vi "Init Device.vi"(8 "error in (no error)":errorcluster, 11 "Toggle 8 in":refnum<class "Toggle 8.lvclass">) -> (0 "error out":errorcluster, 3 "Toggle 8 out":refnum<class "Toggle 8.lvclass">)   [LabVIEW 2020, in "Toggle 8.lvclass"]
doc: "Init the device com port.\nThis should be called by the child class and the child class is responsible for setting the device as its default state."
uses:
  Toggle 8.lvclass
  C:/Sandbox/RF Bench/Source Code/WiSpry Test Framework/Devices/Device.lvclass
  PIC-device/PIC-Device.lvclass
  <instrlib>/Keithley 24XX/Keithley 24XX.lvlib
panel:
  out "Horizontal Graduated Bar":u8(slide) scale=0.0..100.0
  out "Cycle":i32=1
  in  "Stop Button":bool
  # "Beam cycling"
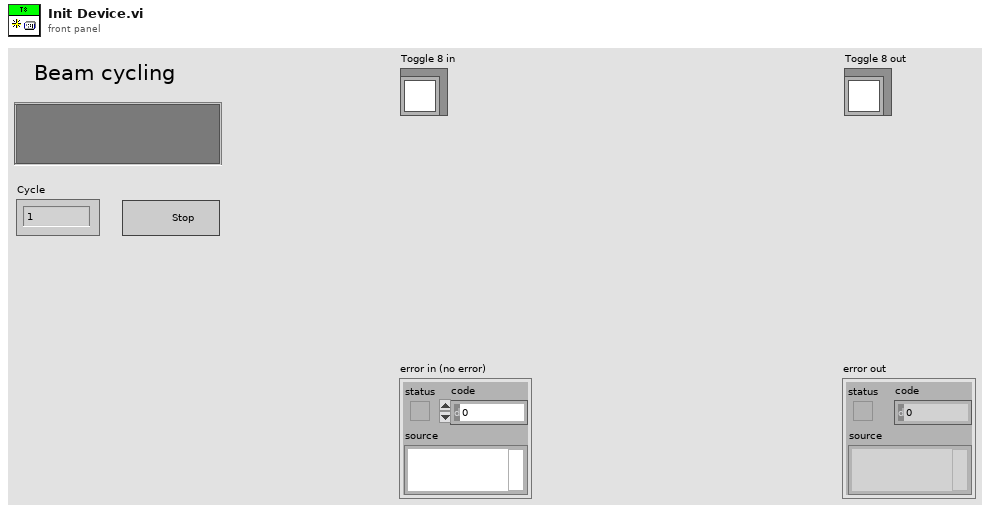
[diagram p1: front panel]
types:
  T1 = enum16{"RFFE 2-wire", "WiSPI 3-wire spi_sel", "WiSPI 4-wire spi_sel", "ifxSPI 3-wire spi_sel", "WiSPI 3-wire dev add spi_sel"}
  T2 = typedef "PIC-Device.lvclass/Register to Write.ctl" = cluster{"Register":u32, "Value":u32, "Dev Address":u32, "Physical Adress":u32}
  T3 = typedef "Toggle 8.lvclass/Test Sequence.ctl" = cluster{"CP values":string, "Charge Pump values":enum16{"CP 24V", "CP 26V", "CP 28V", "CP 30V", "CP 31V", "CP 32V", "CP 33V", "CP 34V", "CP 35V", "CP 36V", "CP 37V", "CP 38V", "CP 39V", "CP 40V", "CP 41V", "CP 42V", "CP 43V", "CP 44V", "CP 45V", "CP 46V", "CP 47V", "CP 48V", "CP 49V", "CP 50V", "CP 51V", "CP 52V", "CP 53V", "CP 54V", "CP 56V", "CP 58V", "CP 60V", "CP 62V"}[], "Charge Pump":T2[], "Control individual beams":bool, "OTP/beam values":dbl[], "Capa settings":T2[], "OTP Values string":string}
  T4 = typedef "Device.lvclass/Device Information Cluster.ctl" = cluster{"Device Info":string[][], "Default Values":T2[], "Fetched info":string[][]}
  T5 = cluster{"Enable":bool, "User init values":string}
  T6 = cluster{"Cycle":bool, "Number of cycles":u32, "Cycles Executed":u32}
  T7 = enum32{"Invalid", "Standard", "Closed", "Hidden", "Minimized", "Maximized"}
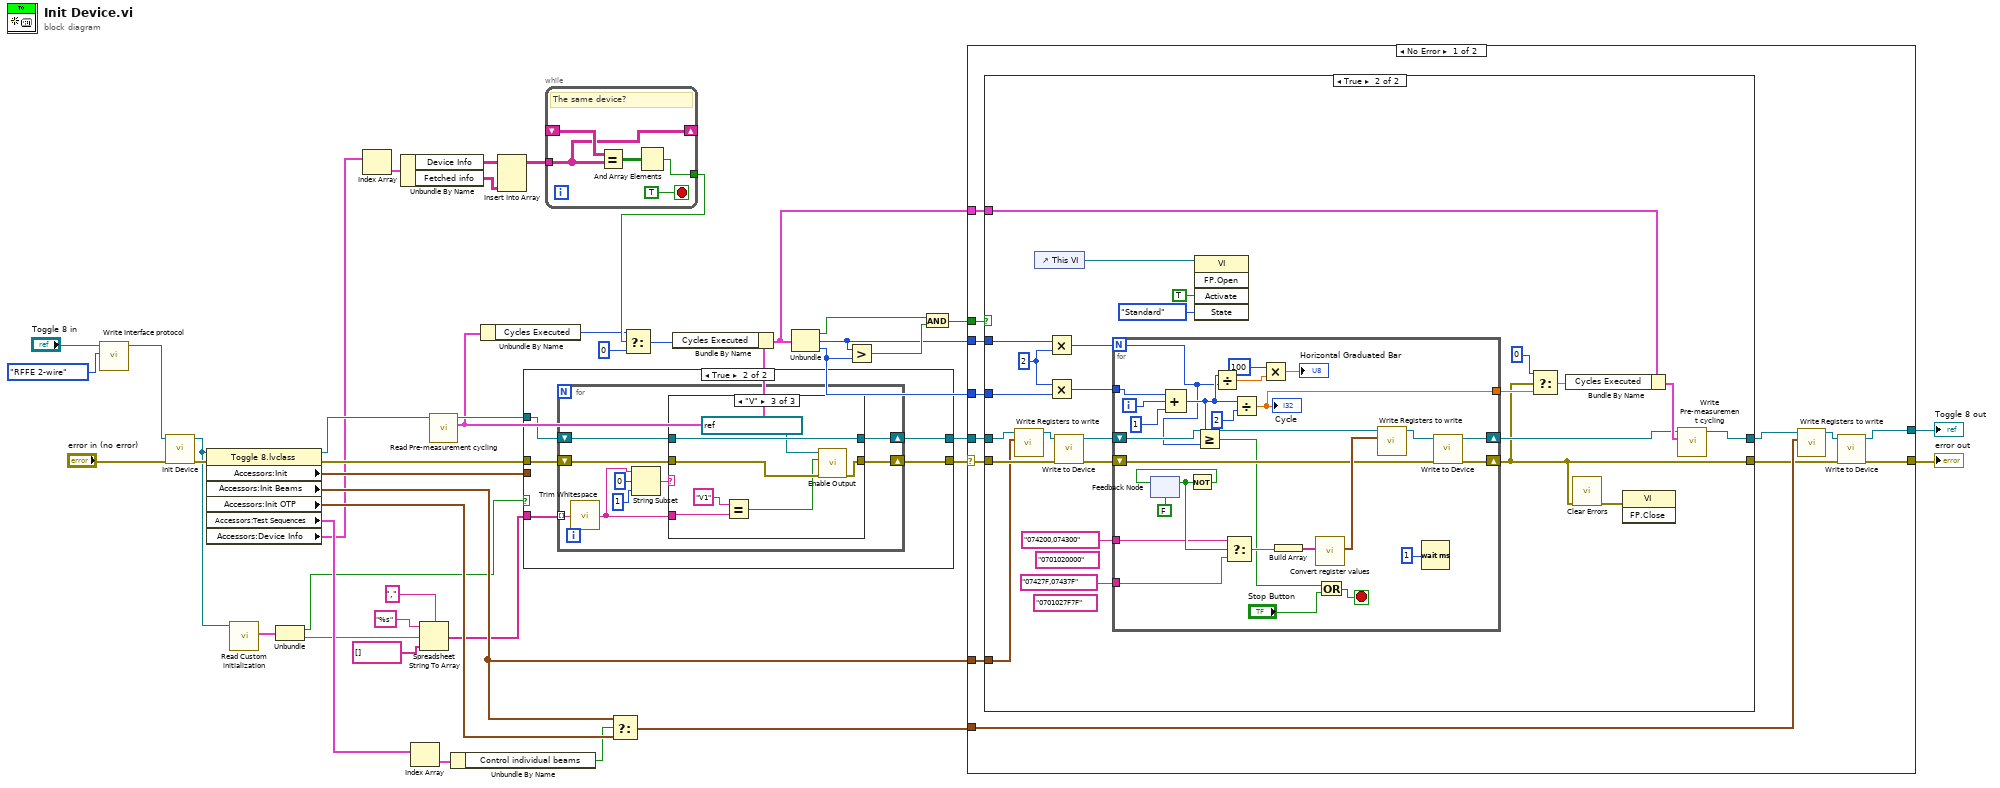
[diagram p0: block diagram]
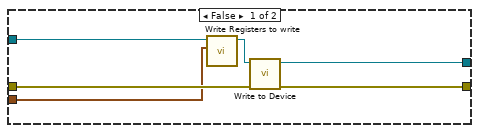
[diagram p2: hidden frame]
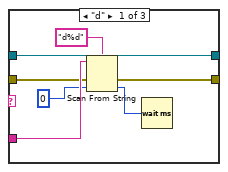
[diagram p3: hidden frame]
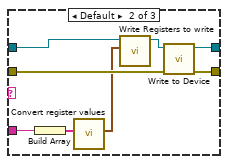
[diagram p4: hidden frame]
diagram:
  n1 = call-dynamic "Write Interface protocol.vi"("Interface protocol"=T1."RFFE 2-wire", "Device in"="Toggle 8 in") -> ("Device out"=w40:refnum<class "Toggle 8.lvclass">)  [unwired: 9 in]
  n2 = call-parent "Init Device.vi"("error in (no error)"="error in (no error)", "Device in"=w40) -> ("error out"=w38:errorcluster, "Device out"=w8:refnum<class "Toggle 8.lvclass">)  [unwired: 8 in]
  n3 = property class="Toggle 8.lvclass"(reference=w8, error in=w38) -> (reference out=w34:refnum<class "Toggle 8.lvclass">, error out=w39:errorcluster, "Accessors:Init"=w26:T2[], "Accessors:Init Beams"=w25:T2[], "Accessors:Init OTP"=w35:T2[], "Accessors:Test Sequences"=w37:T3[], "Accessors:Device Info"=w19:T4[])
  n4 = call-dynamic "Read Custom initialization.vi"("Toggle 8 in"=w8) -> ("Custom initialization"=w7:T5)  [unwired: 9 in, 1 out]
  n5 = Unbundle(w7) -> ("Enable"=w2:bool, "User init values"=w6:string)
  n6 = Index Array(array=w19) -> (element=w18:T4)  [unwired: 1 in]
  n7 = Unbundle By Name(w18) -> ("Device Info"=w11:string[][], "Fetched info"=w9:string[][])
  n8 = Index Array(array=w37) -> (element=w36:T3)  [unwired: 1 in]
  n9 = Spreadsheet String To Array(delimiter (Tab)=",", format string="%s", spreadsheet string=w6, array type (2D Dbl)=string[] []) -> (array=w1:string[])
  n10 = call-dynamic "Read Pre-measurement cycling.vi"("PIC-Device in"=w34) -> ("Pre-measurement cycling"=w16:T6, "PIC-Device out"=w33:refnum<class "Toggle 8.lvclass">)  [unwired: 9 in]
  n11 = Unbundle By Name(w36) -> ("Control individual beams"=w32:bool)
  n12 = Unbundle By Name(w16) -> ("Cycles Executed"=w14:u32)
  n13 = Insert Into Array(array=w11, new element=w9) -> (w10:string[][])  [unwired: 2 in]
  n14 = case shown="True" w2 {
    tunnel: w39 -> [w48 w54]
    tunnel: w33 -> [w47 w53]
    tunnel: [w46 w52] -> w31
    tunnel: [w45 w51] -> w30
    tunnel: w26 -> [w44 _]
    tunnel: w1 -> [_ w50]
    frame False {
      n15 = call-dynamic "Write Registers to write.vi"("Registers to write"=w44, "Device in"=w47) -> ("Device out"=w49:refnum<class "Toggle 8.lvclass">)  [unwired: 9 in]
      n16 = call-dynamic "Write to Device.vi"("error in (no error)"=w48, "Device in"=w49) -> ("error out"=w45:errorcluster, "Device out"=w46:refnum<class "Toggle 8.lvclass">)  [unwired: 7 in, 1 out]
    }
    frame True {
      n17 = for {
        shift-right: [w60] -> w51
        shift-left: w54 -> [w63]
        shift-right: [w61] -> w52
        shift-left: w53 -> [w62]
        tunnel: w50 -> [w56] mode=indexing
        n18 = call <vilib>:"Trim Whitespace.vi"("string"=w56) -> ("trimmed string"=w55:string)  [unwired: 1 in]
        n19 = String Subset(string=w55, offset (0)=0, length (rest)=1 ("length (rest)")) -> (substring=w59:string)
        n20 = case shown="\"V\"" w59 {
          tunnel: w63 -> [w68 w77 w82]
          tunnel: w62 -> [w70 w76 w83]
          tunnel: [w70 w75 w83] -> w61
          tunnel: [w67 w74 w81] -> w60
          tunnel: w55 -> [w69 w73 w85]
          frame "d" {
            n21 = Scan From String(format string="d%d", input string=w69, error in=w68, default 1=u32 0 ("milliseconds to wait")) -> (error out=w67:errorcluster, output 1=w65:u32)  [unwired: 1 in, 2 out]
            n22 = Wait (ms)(milliseconds to wait=w65) -> ()  [unwired: 1 out]
          }
          frame Default {
            n23 = Build Array(w73) -> (w72:string[])
            n24 = call "Convert register values.vi"("Register strings"=w72) -> ("Register clusters out"=w71:T2[])  [unwired: 9 in, 1 out]
            n25 = call-dynamic "Write Registers to write.vi"("Registers to write"=w71, "Device in"=w76) -> ("Device out"=w78:refnum<class "Toggle 8.lvclass">)  [unwired: 9 in]
            n26 = call-dynamic "Write to Device.vi"("error in (no error)"=w77, "Device in"=w78) -> ("error out"=w74:errorcluster, "Device out"=w75:refnum<class "Toggle 8.lvclass">)  [unwired: 7 in, 1 out]
          }
          frame "V" {
            n27 = Equal?(x="V1", y=w85) -> (x = y?=w79:bool)
            n28 = call <instrlib>:"Enable Output.vi"("error in (no error)"=w82, "Enable Output (T: Enable)"=w79, "VISA resource name"=refnum<visa-resource-name> "GPIB0::3::INSTR") -> ("error out"=w81:errorcluster)  [unwired: 7 in, 1 out]
          }
        }
      }
    }
  }
  n29 = while {
    shift-right: [w86] -> _
    shift-left: _ -> [w89]
    tunnel: [w87] -> w15
    tunnel: w10 -> [w86]
    stop <- TRUE stop-if-true
    # "The same device?"
    n30 = Equal?(x=w89, y=w86) -> (x = y?=w88:bool[][])
    n31 = And Array Elements(Boolean array=w88) -> (logical AND=w87:bool)
  }
  n32 = Select(t=w25, s=w32, f=w35) -> (s? t:f=w24:T2[])
  n33 = Select(t=w14, s=w15, f=u32 0) -> (s? t:f=w13:u32)
  n34 = Bundle By Name(cluster=w16, "Cycles Executed"=w13) -> (w17:T6)
  n35 = Unbundle(w17) -> ("Cycle"=w28:bool, "Number of cycles"=w21:u32, "Cycles Executed"=w20:u32)
  n36 = Greater?(x=w21, y=w20) -> (0:w29:bool)
  n37 = And(x=w28, y=w29) -> (x .and. y?=w27:bool)
  n38 = case shown="No Error" w30 {
    selector: w30 -> [w102 w159]
    tunnel: w31 -> [w103 w158]
    tunnel: w27 -> [w101 _]
    tunnel: w25 -> [w99 _]
    tunnel: w24 -> [w98 _]
    tunnel: [w95 w159] -> w23
    tunnel: [w94 w158] -> w22
    tunnel: w21 -> [w93 _]
    tunnel: w20 -> [w92 _]
    tunnel: w17 -> [w91 _]
    frame No Error {
      n39 = case shown="True" w101 {
        tunnel: w103 -> [w104 w116]
        tunnel: [w104 w118] -> w97
        tunnel: [w105 w110] -> w96
        tunnel: w102 -> [w105 w114]
        tunnel: w93 -> [_ w125]
        tunnel: w91 -> [_ w124]
        tunnel: w99 -> [_ w112]
        tunnel: w92 -> [_ w108]
        frame False {
        }
        frame True {
          (unwired) "0701027F7F" ("Write reg 2")
          (unwired) "0701020000" ("Write reg 2")
          w106 = u32 2 ("y")
          n40 = call-dynamic "Write Registers to write.vi"("Registers to write"=w112, "Device in"=w116) -> ("Device out"=w117:refnum<class "Toggle 8.lvclass">)  [unwired: 9 in]
          n41 = control-ref of="This VI"() -> (w128:refnum<vi>)
          n42 = Multiply(x=w125, y=w106) -> (x*y=w109:u32)
          n43 = Multiply(x=w106, y=w108) -> (x*y=w107:u32)
          n44 = call-dynamic "Write to Device.vi"("error in (no error)"=w114, "Device in"=w117) -> ("error out"=w113:errorcluster, "Device out"=w115:refnum<class "Toggle 8.lvclass">)  [unwired: 7 in, 1 out]
          n45 = for {
            N: w109 -> [w132]
            shift-right: [w139] -> w110
            shift-left: w113 -> [w144]
            shift-right: [w152] -> w119
            shift-left: w115 -> [w150]
            tunnel: "074200,074300" ("Write reg 2") -> [w146]
            tunnel: "07427F,07437F" ("Write reg 2") -> [w145]
            tunnel: [w138] -> w121
            tunnel: w107 -> [w134]
            i -> [w149]
            stop <- w136 stop-if-true
            n46 = feedback #1(FALSE) -> (w148:bool)
            n47 = Compound Arithmetic op=ADD(w134, w149, 1 ("value")) -> (w133:u32)
            n48 = Not(x=w148) -> (.not. x?=w156:bool)
            n49 = feedback-in #1(w156) -> ()
            n50 = Greater Or Equal?(x=w133, y=w132) -> (x >= y?=w131:bool)
            n51 = Divide(x=w133, y=w132) -> (x/y=w143:dbl)
            n52 = Select(t=w146, s=w148, f=w145) -> (s? t:f=w151:string)
            n53 = Divide(x=w133, y=2) -> (x/y=w138:dbl)
            "Cycle" <- w138
            n54 = Multiply(x=100, y=w143) -> (x*y=→"Horizontal Graduated Bar":dbl)
            n55 = Build Array(w151) -> (w153:string[])
            n56 = call "Convert register values.vi"("Register strings"=w153) -> ("Register clusters out"=w154:T2[])  [unwired: 9 in, 1 out]
            n57 = Or(x=w131, y="Stop Button") -> (x .or. y?=w136:bool)
            n58 = call-dynamic "Write Registers to write.vi"("Registers to write"=w154, "Device in"=w150) -> ("Device out"=w155:refnum<class "Toggle 8.lvclass">)  [unwired: 9 in]
            n59 = Wait (ms)(milliseconds to wait=u32 1) -> ()  [unwired: 1 out]
            n60 = call-dynamic "Write to Device.vi"("error in (no error)"=w144, "Device in"=w155) -> ("error out"=w139:errorcluster, "Device out"=w152:refnum<class "Toggle 8.lvclass">)  [unwired: 7 in, 1 out]
          }
          n61 = invoke class="VI" method="FP.Open"(reference=w128, "Activate"=TRUE ("Activate?"), "State"=T7."Standard") -> ()  [unwired: 2 in, 5 out]
          n62 = Select(t=0 ("x"), s=w110, f=w121) -> (s? t:f=w122:dbl)
          n63 = Bundle By Name(cluster=w124, "Cycles Executed"=w122) -> (w123:T6)
          n64 = call <vilib>:"Clear Errors.vi"("error in (no error)"=w110) -> ("error out"=w111:errorcluster)  [unwired: 5 in, 1 out]
          n65 = invoke class="VI" method="FP.Close"(error in=w111) -> ()  [unwired: 2 in, 3 out]
          n66 = call-dynamic "Write Pre-measurement cycling.vi"("Pre-measurement cycling"=w123, "PIC-Device in"=w119) -> ("PIC-Device out"=w118:refnum<class "Toggle 8.lvclass">)  [unwired: 9 in]
        }
      }
      n67 = call-dynamic "Write Registers to write.vi"("Registers to write"=w98, "Device in"=w97) -> ("Device out"=w100:refnum<class "Toggle 8.lvclass">)  [unwired: 9 in]
      n68 = call-dynamic "Write to Device.vi"("error in (no error)"=w96, "Device in"=w100) -> ("error out"=w95:errorcluster, "Device out"=w94:refnum<class "Toggle 8.lvclass">)  [unwired: 7 in, 1 out]
    }
    frame Error {
    }
  }
  "error out" <- w23
  "Toggle 8 out" <- w22
